vi "SA_RAD_STD.vi"(4 "RO":bool, 6 "RAD STD":i32(ring) items=["NONE", "GSM"], 8 "error in":errorcluster {"code" format="%.0x"}, 11 "Session In":refnum<visa-resource-name>="TCPIP0::K-N90X0A-00005.local::hislip0::INSTR") -> (0 "error out":errorcluster {"code" format="%.0x"}, 3 "Session Out":refnum<visa-resource-name>, 5 "rad std":string)   [LabVIEW 2018]
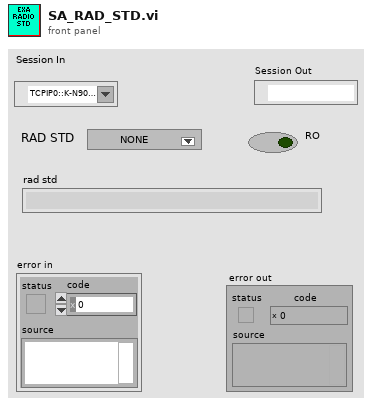
[diagram p1: front panel]
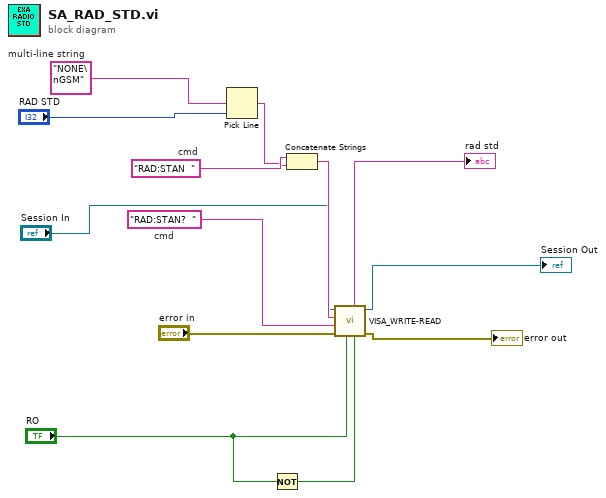
[diagram p0: block diagram]
diagram:
  w6 = "RAD:STAN?  "  # cmd
  w9 = "RAD:STAN  "  # cmd
  w13 = "NONE\nGSM"  # multi-line string
  n1 = Pick Line(multi-line string=w13, line index="RAD STD") -> (output string=w8:string)  [unwired: 1 in]
  n2 = Not(x="RO") -> (.not. x?=w1:bool)
  n3 = Concatenate Strings(w9, w8) -> (w7:string)
  n4 = call "VISA_WRITE-READ.vi"("WRITE"=w1, "READ"="RO", "error in"="error in", "Rcmd"=w6, "Wcmd"=w7, "Session In"="Session In") -> ("error out"=→"error out":errorcluster, "Session Out"=→"Session Out":refnum<visa-resource-name>, "Out"=→"rad std":string)  [unwired: 3 in]
